vi "move_and_extract_roi.vi"(8 "error in (no error)":errorcluster, 10 "Change in ROI":i32[](array[numeric]), 11 "Image Ctl":refnum<vi>) -> (0 "error out":errorcluster, 1 "Old Global Rectangle":i32[](array[numeric]), 2 "Rectangles":i32[][](array[numeric]), 3 "Image Ctl Dup":refnum<vi>)   [LabVIEW 2010]
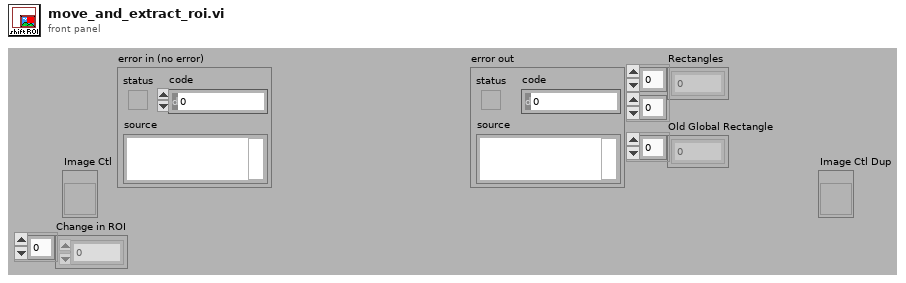
[diagram p1: front panel]
types:
  T1 = cluster{"Global Rectangle":i32[], "Contours":cluster{"Contour Type":u32, "ROI Type":u32, "Points":i32[]}[]}
  T2 = cluster{"Contour Type":u32, "ROI Type":u32, "Points":i32[]}[]
  T3 = cluster{"Contour Type":u32, "ROI Type":u32, "Points":i32[]}
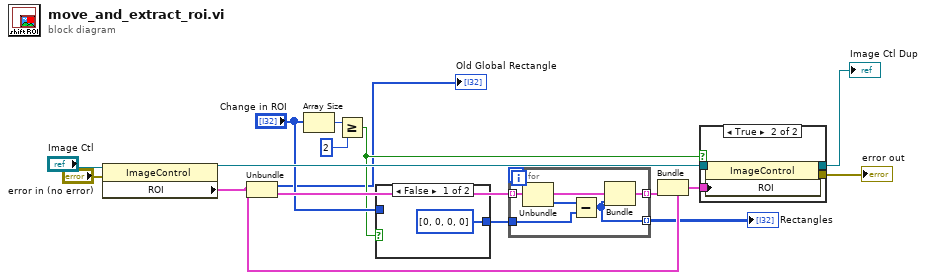
[diagram p0: block diagram]
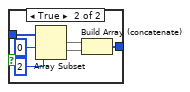
[diagram p3: hidden frame]
diagram:
  n1 = property on="Property Node" class="ImageControl"(reference="Image Ctl", error in="error in (no error)") -> (reference out=w11:refnum<vi>, "ROI"=w14:T1)  [unwired: 1 out]
  n2 = Unbundle(w14) -> ("Global Rectangle"=→"Old Global Rectangle":i32[], "Contours"=w16:T2)
  n3 = Array Size(array="Change in ROI") -> (size(s)=w4:i32)
  n4 = Greater Or Equal?(x=w4, y=2) -> (x >= y?=w2:bool)
  n5 = case shown="False" w2 {
    tunnel: [i32[] [0, 0, 0, 0] w19] -> w15
    tunnel: "Change in ROI" -> [_ w18]
    frame False {
    }
    frame True {
      n6 = Array Subset(array=w18, index=0, length=2) -> (w20:i32[])
      n7 = Build Array (concatenate)(w20, w20) -> (w19:i32[])
    }
  }
  n8 = for {
    tunnel: w16 -> [w25] mode=indexing
    tunnel: w15 -> [w26]
    tunnel: [w24] -> w13 mode=indexing
    tunnel: [w23] -> w6 mode=indexing
    n9 = Unbundle(w25) -> ("Points"=w27:i32[])  [unwired: 2 out]
    n10 = Subtract(x=w27, y=w26) -> (x-y=w23:i32[])
    n11 = Bundle(cluster=w25, "Points"=w23) -> (w24:T3)  [unwired: 2 in]
  }
  "Rectangles" <- w6
  n12 = Bundle(cluster=w14, "Contours"=w13) -> (w12:T1)  [unwired: 1 in]
  n13 = case shown="True" w2 {
    tunnel: w12 -> [_ w32]
    tunnel: w11 -> [w28 w31]
    tunnel: [_ w30] -> w8
    tunnel: [w28 w29] -> w7
    frame False {
    }
    frame True {
      n14 = property on="Property Node" class="ImageControl"(reference=w31, "ROI"=w32) -> (reference out=w29:refnum<vi>, error out=w30:errorcluster)  [unwired: 1 in]
    }
  }
  "Image Ctl Dup" <- w7
  "error out" <- w8
